vi "Open-Create-Replace File.vi"(4 "advisory dialog? (display:T)":bool=TRUE, 5 "pattern":string, 6 "default name":string, 7 "prompt":string, 8 "error in (no error)":errorcluster, 9 "function (open:0)":T2(ring), 10 "start path  (Not A Path)":path=path "", 11 "file path":path) -> (0 "error out":errorcluster, 1 "file size (bytes)":i32, 2 "new file path":path, 3 "refnum":refnum<file>)   [LabVIEW 2009]
doc: "Opens an existing file, creates a new file, or replaces an existing file, programmatically or interactively using a file dialog box."
panel:
  in  "Messages":T1={"Replace existing \"%s\"?"="Replace existing \"%s\"?", "File \"%s\" exists."="File \"%s\" exists.", "Cancel"="Cancel", "Replace"="Replace", "\"%s\" not found."="\"%s\" not found.", "Open File"="Open File", "New File"="New File", "Create File (file exists)"="Create File (file exists)", "File Dialog"="File Dialog", "Open or Create File %d"="Open or Create File (function=%d)", "EOF"="EOF"}
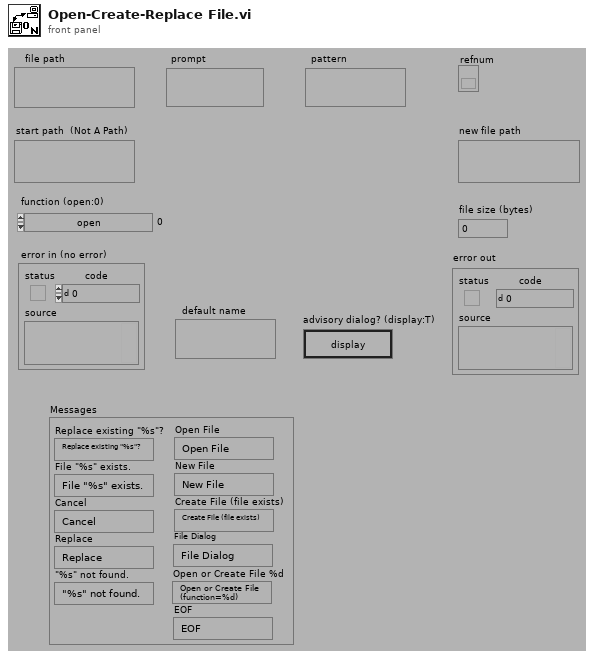
[diagram p1: front panel]
types:
  T1 = cluster{"Replace existing \"%s\"?":string, "File \"%s\" exists.":string, "Cancel":string, "Replace":string, "\"%s\" not found.":string, "Open File":string, "New File":string, "Create File (file exists)":string, "File Dialog":string, "Open or Create File %d":string, "EOF":string}
  T2 = enum16{"open", "open or create", "create or replace", "create", "open (read only)"}
  T3 = enum16{"read/write", "read-only", "write-only", "write-only (truncate)"}
  T4 = enum16{"open", "open or create", "create or replace", "create"}
  T5 = enum16{"open", "replace", "create", "open or create", "replace or create", "replace or create with confirmation"}
  T6 = enum16{"existing file", "new file", "new or existing file", "existing dir", "new dir", "new or existing dir"}[]
  T7 = enum16{"existing file", "new file", "new or existing file", "existing dir", "new dir", "new or existing dir"}
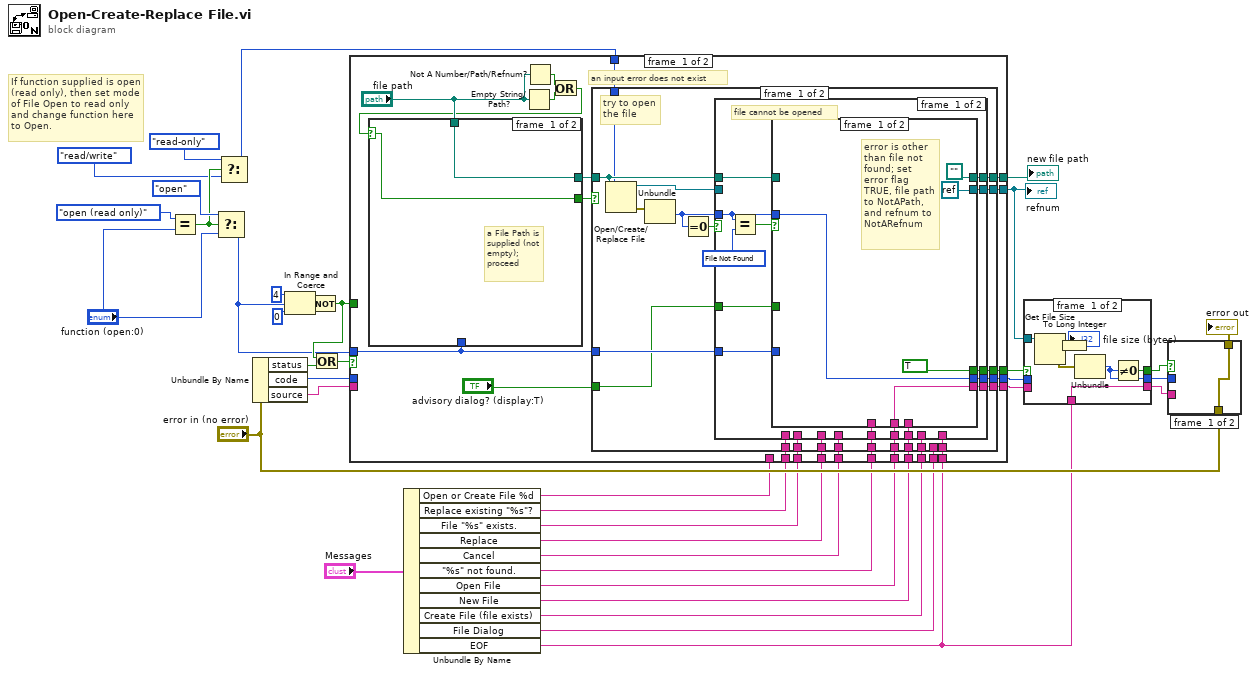
[diagram p0: block diagram]
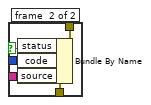
[diagram p2: hidden frame]
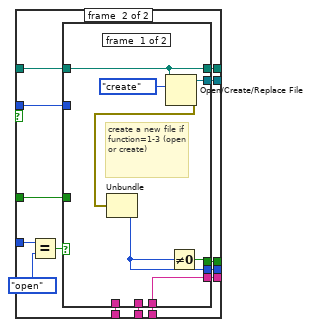
[diagram p4: hidden frame]
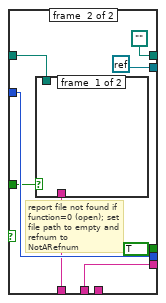
[diagram p5: hidden frame]
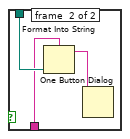
[diagram p6: hidden frame]
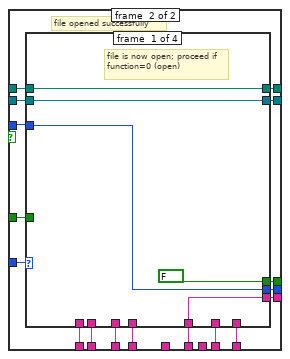
[diagram p7: hidden frame]
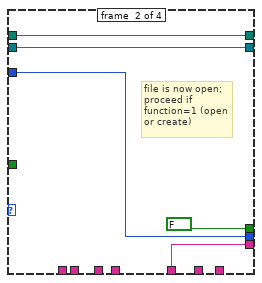
[diagram p8: hidden frame]
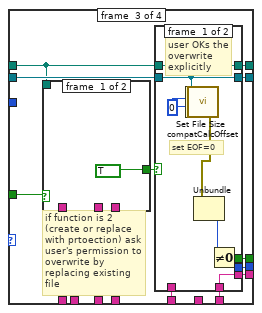
[diagram p9: hidden frame]
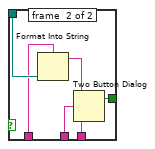
[diagram p10: hidden frame]
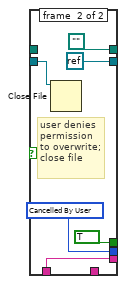
[diagram p11: hidden frame]
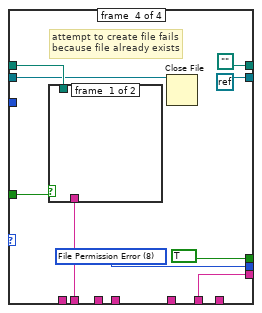
[diagram p12: hidden frame]
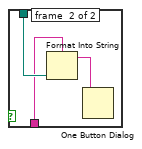
[diagram p13: hidden frame]
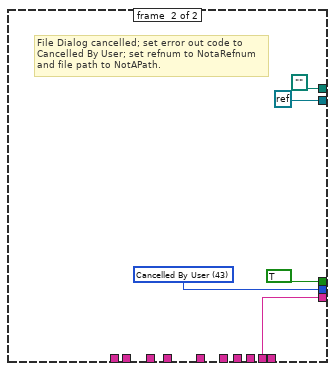
[diagram p14: hidden frame]
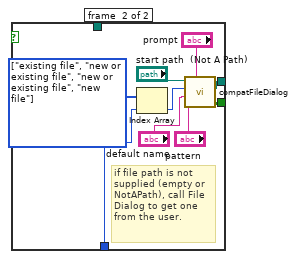
[diagram p15: hidden frame]
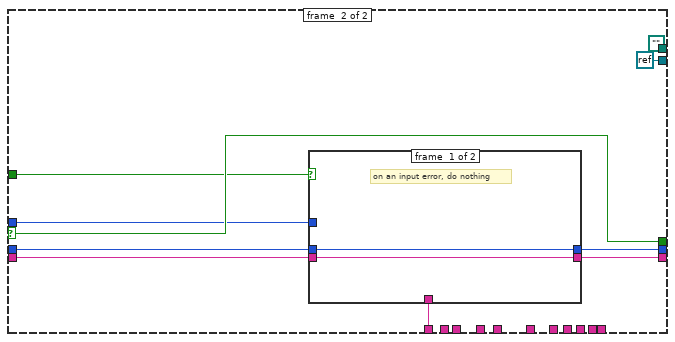
[diagram p16: hidden frame]
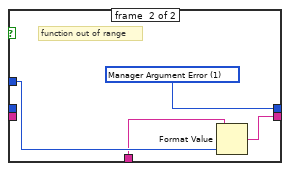
[diagram p17: hidden frame]
diagram:
  # "If function supplied is open (read only), then set mode of File Open to read only and change function here to Open."
  n1 = Equal?(x=T2."open (read only)" ("y"), y="function (open:0)") -> (x = y?=w6:bool)
  n2 = Select(t=T2."open", s=w6, f="function (open:0)") -> (s? t:f=w3:T2)
  n3 = Select(t=T3."read-only" ("open mode (0)"), s=w6, f=T3."read/write" ("open mode (0)")) -> (s? t:f=w1:T3)
  n4 = Unbundle By Name("error in (no error)") -> ("status"=w28:bool, "code"=w27:i32, "source"=w26:string)
  n5 = In Range and Coerce(upper limit=4, x=w3, lower limit=0) -> (In Range?=w33:bool)  [unwired: 1 out]
  n6 = Not(x=w33) -> (.not. x?=w35:bool)
  n7 = Or(x=w35, y=w28) -> (x .or. y?=w34:bool)
  n8 = Unbundle By Name("Messages") -> ("Open or Create File %d"=w10:string, "Replace existing \"%s\"?"=w19:string, "File \"%s\" exists."=w18:string, "Replace"=w17:string, "Cancel"=w16:string, "\"%s\" not found."=w15:string, "Open File"=w14:string, "New File"=w13:string, "Create File (file exists)"=w12:string, "File Dialog"=w11:string, "EOF"=w9:string)
  n9 = case shown="False" w34 {
    selector: w34 -> [_ w235]
    tunnel: [w60 path ""] -> w38
    tunnel: [w59 refnum<k0> refnum] -> w29
    tunnel: [w58 w232] -> w30
    tunnel: [w57 w235] -> w32
    tunnel: [w56 w234] -> w31
    tunnel: w27 -> [_ w233]
    tunnel: w26 -> [_ w231]
    tunnel: w3 -> [w50 w230]
    tunnel: w35 -> [_ w229]
    tunnel: w14 -> [w49 _]
    tunnel: w13 -> [w48 _]
    tunnel: w15 -> [w47 _]
    tunnel: w16 -> [w46 _]
    tunnel: w17 -> [w45 _]
    tunnel: w19 -> [w44 _]
    tunnel: w12 -> [w43 _]
    tunnel: w18 -> [w42 _]
    tunnel: w11 -> [w41 _]
    tunnel: w10 -> [_ w228]
    tunnel: w9 -> [w40 _]
    tunnel: w1 -> [w39 _]
    frame #0 {
      # "an input error does not exist"
      n10 = Empty String/Path?(string/path="file path") -> (empty?=w53:bool)
      n11 = Not A Number/Path/Refnum?(number/path/refnum="file path") -> (NaN/Path/Refnum?=w54:bool)
      n12 = Or(x=w54, y=w53) -> (x .or. y?=w52:bool)
      n13 = case shown="True" w52 {
        selector: w52 -> [w217 _]
        tunnel: [w217 w225] -> w62
        tunnel: [w218 w224] -> w61
        tunnel: "file path" -> [w218 _]
        tunnel: w50 -> [_ w220]
        frame #0 {
          # "a File Path is supplied (not empty); proceed"
        }
        frame #1 {
          w221 = T6 [enum."existing file", enum."new or existing file", enum."new or existing file", enum."new file"] items=["existing file", "new file", "new or existing file", "existing dir", "new dir", "new or existing dir"]
          # "if file path is not supplied (empty or NotAPath), call File Dialog to get one from the user."
          n14 = Index Array(array=w221, index=w220) -> (element=w222:T7)
          n15 = call <vilib>:"compatFileDialog.vi"("prompt"="prompt", "pattern"="pattern", "default name"="default name", "select mode (2)"=w222, "start path"="start path  (Not A Path)") -> ("cancelled"=w225:bool, "path"=w224:path)  [unwired: 4 in, 1 out]
        }
      }
      n16 = case shown="False" w62 {
        tunnel: w61 -> [w83 _]
        tunnel: [w82 path ""] -> w60
        tunnel: w50 -> [w81 _]
        tunnel: [w80 refnum<k0> refnum] -> w59
        tunnel: [w78 w212] -> w58
        tunnel: [w77 TRUE] -> w57
        tunnel: [w76 w215] -> w56
        tunnel: "advisory dialog? (display:T)" -> [w74 _]
        tunnel: w49 -> [w72 _]
        tunnel: w48 -> [w71 _]
        tunnel: w47 -> [w70 _]
        tunnel: w46 -> [w69 _]
        tunnel: w45 -> [w68 _]
        tunnel: w44 -> [w67 _]
        tunnel: w43 -> [w66 _]
        tunnel: w42 -> [w65 _]
        tunnel: w41 -> [_ w212]
        tunnel: w40 -> [w64 _]
        tunnel: w39 -> [w63 _]
        frame #0 {
          # "try to open the file"
          n17 = Open/Create/Replace File(file path (use dialog)=w83, access (0:read/write)=w63) -> (refnum out=w79:refnum<file>, error out=w84:errorcluster)  [unwired: 4 in, 1 out]
          n18 = Unbundle(w84) -> ("code"=w73:i32)  [unwired: 2 out]
          n19 = Equal To 0?(x=w73) -> (x = 0?=w75:bool)
          n20 = case shown="True" w75 {
            tunnel: w73 -> [w89 w145]
            tunnel: w83 -> [w96 w151]
            tunnel: [w95 w152] -> w82
            tunnel: w81 -> [w94 w144]
            tunnel: [w93 w150] -> w80
            tunnel: w79 -> [_ w149]
            tunnel: [w92 w148] -> w78
            tunnel: [w91 w147] -> w77
            tunnel: [w90 w146] -> w76
            tunnel: w74 -> [w88 w143]
            tunnel: w72 -> [w87 w142]
            tunnel: w71 -> [w86 _]
            tunnel: w70 -> [w85 _]
            tunnel: w69 -> [_ w141]
            tunnel: w68 -> [_ w140]
            tunnel: w67 -> [_ w139]
            tunnel: w66 -> [_ w138]
            tunnel: w65 -> [_ w137]
            tunnel: w64 -> [_ w136]
            frame #0 {
              w98 = u16 7 items=["No Error", "Manager Argument Error", "Memory Full", "Out of Zone", "End of File", "File Already Open", "Generic File IO Error", "File Not Found", "File Permission Error", "Disk Full", "Duplicate Path", "Too Many Files Open", "Not Enabled", "Resource File Not Found", "Cannot Add Resource", "Resource Not Found", "Image Not Found", "Image Memory Error", "Pen Does Not Exist", "Config Bad Type", "Config Token Not Found", "Config Parse Error", "Config Memory Error", "Bad External Code Format", "Bad External Code Offset", "External Code Not Present", "Null Window", "Destroy Window Mixup", "Null Menu", "Print Aborted", "Bad Print Record", "Print Driver Error", "Windows Error During Print", "Memory Error During Print", "Print Dialog Error", "Generic Print Error", "Invalid Device Refnum", "Device Not Found", "Device Parameter Error", "Device Unit Error", "Can't Open Device", "Device Call Aborted", "Generic Error", "Cancelled By User"]
              # "file cannot be opened"
              n21 = Equal?(x=w89, y=w98) -> (x = y?=w97:bool)
              n22 = case shown="True" w97 {
                tunnel: w96 -> [_ w117]
                tunnel: [path "" w116] -> w95
                tunnel: w94 -> [_ w109]
                tunnel: [refnum<k0> refnum w115] -> w93
                tunnel: [w99 w114] -> w92
                tunnel: [TRUE w113] -> w91
                tunnel: [w100 w112] -> w90
                tunnel: w89 -> [w100 w111]
                tunnel: w88 -> [_ w110]
                tunnel: w87 -> [w99 w105]
                tunnel: w86 -> [_ w106]
                tunnel: w85 -> [_ w104]
                frame #0 {
                  # "error is other than file not found; set error flag TRUE, file path to NotAPath, and refnum to NotARefnum"
                }
                frame #1 {
                  n23 = Equal?(x=w109, y=T4."open") -> (x = y?=w108:bool)
                  n24 = case shown="True" w108 {
                    tunnel: w117 -> [w124 w130]
                    tunnel: [w124 path ""] -> w116
                    tunnel: [w123 refnum<k0> refnum] -> w115
                    tunnel: [w119 w126] -> w114
                    tunnel: [w122 TRUE] -> w113
                    tunnel: [w120 w131] -> w112
                    tunnel: w111 -> [_ w131]
                    tunnel: w110 -> [_ w127]
                    tunnel: w106 -> [w119 _]
                    tunnel: w105 -> [_ w126]
                    tunnel: w104 -> [_ w125]
                    frame #0 {
                      # "create a new file if function=1-3 (open or create)"
                      n25 = Open/Create/Replace File(file path (use dialog)=w124, operation (0:open)=T5."create") -> (refnum out=w123:refnum<file>, error out=w121:errorcluster)  [unwired: 4 in, 1 out]
                      n26 = Unbundle(w121) -> ("code"=w120:i32)  [unwired: 2 out]
                      n27 = Not Equal To 0?(x=w120) -> (x != 0?=w122:bool)
                    }
                    frame #1 {
                      # "report file not found if function=0 (open); set file path to empty and refnum to NotARefnum"
                      n28 = case shown="True" w127 {
                        tunnel: w130 -> [_ w135]
                        tunnel: w125 -> [_ w134]
                        frame #0 {
                        }
                        frame #1 {
                          n29 = Format Into String(format string=w134, w135) -> (resulting string=w133:string)  [unwired: 2 in, 1 out]
                          n30 = One Button Dialog(message=w133) -> ()  [unwired: 1 in, 1 out]
                        }
                      }
                    }
                  }
                }
              }
            }
            frame #1 {
              # "file opened successfully"
              n31 = case shown="\"create or replace\"" w144 {
                tunnel: [w157 w159 w176 path ""] -> w152
                tunnel: w151 -> [w157 w159 w168 w208]
                tunnel: [w156 w160 w175 refnum<k0> refnum] -> w150
                tunnel: w149 -> [w156 w160 w174 w205]
                tunnel: [w153 w158 w173 w201] -> w148
                tunnel: [FALSE FALSE w172 TRUE] -> w147
                tunnel: [w154 w162 w171 w206] -> w146
                tunnel: w145 -> [w154 w162 _ _]
                tunnel: w143 -> [_ _ w169 w207]
                tunnel: w142 -> [w153 w158 w164 _]
                tunnel: w141 -> [_ _ w167 _]
                tunnel: w140 -> [_ _ w166 _]
                tunnel: w139 -> [_ _ w165 _]
                tunnel: w138 -> [_ _ _ w201]
                tunnel: w137 -> [_ _ _ w200]
                tunnel: w136 -> [_ _ w163 _]
                frame #0 {
                  # "file is now open; proceed if function=0 (open)"
                }
                frame #1 {
                  # "file is now open; proceed if function=1 (open or create)"
                }
                frame #2 {
                  # "if function is 2 (create or replace with prtoection) ask user's permission to overwrite by replacing existing file"
                  n32 = case shown="False" w169 {
                    tunnel: [TRUE w183] -> w170
                    tunnel: w168 -> [_ w180]
                    tunnel: w167 -> [_ w181]
                    tunnel: w166 -> [_ w182]
                    tunnel: w165 -> [_ w178]
                    frame #0 {
                    }
                    frame #1 {
                      n33 = Format Into String(format string=w178, w180) -> (resulting string=w179:string)  [unwired: 2 in, 1 out]
                      n34 = Two Button Dialog(message=w179, 1:w181, 2:w182) -> (T button?=w183:bool)
                    }
                  }
                  n35 = case shown="True" w170 {
                    tunnel: [w189 path ""] -> w176
                    tunnel: [w193 refnum<k0> refnum] -> w175
                    tunnel: w174 -> [w193 w197]
                    tunnel: [w187 w194] -> w173
                    tunnel: [w191 TRUE] -> w172
                    tunnel: [w188 w195] -> w171
                    tunnel: w168 -> [w189 _]
                    tunnel: w164 -> [_ w194]
                    tunnel: w163 -> [w187 _]
                    frame #0 {
                      w192 = 0
                      # "set EOF=0"
                      # "user OKs the overwrite explicitly"
                      n36 = call <vilib>:"compatCalcOffset.vi"("pos offset (0)"=w192, "pos mode (0:1)"=w192, "refnum"=w193) -> ("error out"=w186:errorcluster, "offset"=w185:i32, "dup refnum"=w184:refnum<file>)  [unwired: 6 in]
                      n37 = Set File Size(4:w186, 6:w185, 7:w184) -> (0:w190:errorcluster)  [unwired: 1 out]
                      n38 = Unbundle(w190) -> ("code"=w188:i32)  [unwired: 2 out]
                      n39 = Not Equal To 0?(x=w188) -> (x != 0?=w191:bool)
                    }
                    frame #1 {
                      w195 = u16 43 items=["No Error", "Manager Argument Error", "Memory Full", "Out of Zone", "End of File", "File Already Open", "Generic File IO Error", "File Not Found", "File Permission Error", "Disk Full", "Duplicate Path", "Too Many Files Open", "Not Enabled", "Resource File Not Found", "Cannot Add Resource", "Resource Not Found", "Image Not Found", "Image Memory Error", "Pen Does Not Exist", "Config Bad Type", "Config Token Not Found", "Config Parse Error", "Config Memory Error", "Bad External Code Format", "Bad External Code Offset", "External Code Not Present", "Null Window", "Destroy Window Mixup", "Null Menu", "Print Aborted", "Bad Print Record", "Print Driver Error", "Windows Error During Print", "Memory Error During Print", "Print Dialog Error", "Generic Print Error", "Invalid Device Refnum", "Device Not Found", "Device Parameter Error", "Device Unit Error", "Can't Open Device", "Device Call Aborted", "Generic Error", "Cancelled By User"]
                      # "user denies permission to overwrite; close file"
                      n40 = Close File(refnum=w197) -> ()  [unwired: 1 in, 2 out]
                    }
                  }
                }
                frame #3 {
                  w206 = u16 8 items=["No Error", "Argument Error", "Memory Full", "Out of Zone", "End of File", "File Already Open", "Generic File IO Error", "File Not Found", "File Permission Error", "Disk Full", "Duplicate Path", "Too Many Files Open", "Not Enabled", "Resource File Not Found", "Cannot Add Resource", "Resource Not Found", "Image Not Found", "Image Memory Error", "Pen Does Not Exist", "Config Bad Type", "Config Token Not Found", "Config Parse Error", "Config Memory Error", "Bad External Code Format", "Bad External Code Offset", "External Code Not Present", "Null Window", "Destroy Window Mixup", "Null Menu", "Print Aborted", "Bad Print Record", "Print Driver Error", "Windows Error During Print", "Memory Error During Print", "Print Dialog Error", "Generic Print Error", "Invalid Device Refnum", "Device Not Found", "Device Parameter Error", "Device Unit Error", "Can't Open Device", "Device Call Aborted", "Generic Error", "Cancelled By User", "Object ID Too Low", "Object ID Too High", "Object Not In Heap", "Unknown Heap", "Bad DefProc ID", "DefProc Not In Table", "Message Out Of Range", "Null Method", "Unknown Message", "Manager Call Not Supported", "Bad address", "Connection In progress", "Connection timed out", "Connection is already in progress", "Network attribute not supported", "Network error", "Address in use", "System out of memory", "Connection aborted", "Connection refused", "Connection is not connected", "Connection is already connected", "Connection closed", "Initialize error (interapplication manager)", "Bad occurrence", "Wait on unbound occurrence handler", "Occurrence queue overflow", "Bad path", "Semaphore not signaled", "Unrecognized type (interapplication manager)"]
                  # "attempt to create file fails because file already exists"
                  n41 = case shown="True" w207 {
                    tunnel: w208 -> [_ w211]
                    tunnel: w200 -> [_ w209]
                    frame #0 {
                    }
                    frame #1 {
                      n42 = Format Into String(format string=w209, w211) -> (resulting string=w210:string)  [unwired: 2 in, 1 out]
                      n43 = One Button Dialog(message=w210) -> ()  [unwired: 1 in, 1 out]
                    }
                  }
                  n44 = Close File(refnum=w205) -> ()  [unwired: 1 in, 2 out]
                }
              }
            }
          }
        }
        frame #1 {
          w215 = u16 43 items=["No Error", "Manager Argument Error", "Memory Full", "Out of Zone", "End of File", "File Already Open", "Generic File IO Error", "File Not Found", "File Permission Error", "Disk Full", "Duplicate Path", "Too Many Files Open", "Not Enabled", "Resource File Not Found", "Cannot Add Resource", "Resource Not Found", "Image Not Found", "Image Memory Error", "Pen Does Not Exist", "Config Bad Type", "Config Token Not Found", "Config Parse Error", "Config Memory Error", "Bad External Code Format", "Bad External Code Offset", "External Code Not Present", "Null Window", "Destroy Window Mixup", "Null Menu", "Print Aborted", "Bad Print Record", "Print Driver Error", "Windows Error During Print", "Memory Error During Print", "Print Dialog Error", "Generic Print Error", "Invalid Device Refnum", "Device Not Found", "Device Parameter Error", "Device Unit Error", "Can't Open Device", "Device Call Aborted", "Generic Error", "Cancelled By User"]
          # "File Dialog cancelled; set error out code to Cancelled By User; set refnum to NotaRefnum and file path to NotAPath."
        }
      }
    }
    frame #1 {
      n45 = case shown="True" w229 {
        tunnel: [w239 w243] -> w234
        tunnel: w233 -> [w239 _]
        tunnel: [w238 w242] -> w232
        tunnel: w231 -> [w238 _]
        tunnel: w230 -> [_ w241]
        tunnel: w228 -> [_ w240]
        frame #0 {
          # "on an input error, do nothing"
        }
        frame #1 {
          w243 = u16 1 items=["No Error", "Manager Argument Error", "Memory Full", "Out of Zone", "End of File", "File Already Open", "Generic File IO Error", "File Not Found", "File Permission Error", "Disk Full", "Duplicate Path", "Too Many Files Open", "Not Enabled", "Resource File Not Found", "Cannot Add Resource", "Resource Not Found", "Image Not Found", "Image Memory Error", "Pen Does Not Exist", "Config Bad Type", "Config Token Not Found", "Config Parse Error", "Config Memory Error", "Bad External Code Format", "Bad External Code Offset", "External Code Not Present", "Null Window", "Destroy Window Mixup", "Null Menu", "Print Aborted", "Bad Print Record", "Print Driver Error", "Windows Error During Print", "Memory Error During Print", "Print Dialog Error", "Generic Print Error", "Invalid Device Refnum", "Device Not Found", "Device Parameter Error", "Device Unit Error", "Can't Open Device", "Device Call Aborted", "Generic Error", "Cancelled By User"]
          # "function out of range"
          n46 = Format Value(format string=w240, value (0)=w241) -> (output string=w242:string)  [unwired: 1 in]
        }
      }
    }
  }
  "new file path" <- w38
  "refnum" <- w29
  n47 = case shown="False" w32 {
    selector: w32 -> [_ w253]
    tunnel: w31 -> [_ w252]
    tunnel: w30 -> [_ w251]
    tunnel: [w250 w253] -> w25
    tunnel: [w247 w252] -> w24
    tunnel: [w245 w251] -> w23
    tunnel: w29 -> [w249 _]
    tunnel: w9 -> [w245 _]
    frame #0 {
      n48 = Get File Size(file=w249) -> (size (in bytes)=w244:i64, 0:w246:errorcluster)  [unwired: 1 in, 1 out]
      n49 = To Long Integer(number=w244) -> (32bit integer=→"file size (bytes)":i32)
      n50 = Unbundle(w246) -> ("code"=w247:i32)  [unwired: 2 out]
      n51 = Not Equal To 0?(x=w247) -> (x != 0?=w250:bool)
    }
    frame #1 {
    }
  }
  n52 = case shown="True" w25 {
    selector: w25 -> [_ w258]
    tunnel: w24 -> [_ w259]
    tunnel: w23 -> [_ w257]
    tunnel: "error in (no error)" -> [w254 w256]
    tunnel: [w254 w255] -> w21
    frame #0 {
    }
    frame #1 {
      n53 = Bundle By Name(cluster=w256, "status"=w258, "code"=w259, "source"=w257) -> (w255:errorcluster)
    }
  }
  "error out" <- w21
